vi "BenchmarkSystemDefinition.vi"(4 "Tolerance (%)":dbl=3.0 format="%#_13g", 5 "Duration (s)":dbl=30.0 format="%#_13g", 6 "Gateway IP Address (\"\": localhost)":string, 7 "Target Rate List in":dbl[](array[numeric]), 8 "error in (no error)":errorcluster, 9 "overrides files":path[](array[path]), 10 "System Definition File":path, 11 "VeriStandTestCase in":refnum<class "VeriStandTestCase.lvclass">) -> (0 "error out":errorcluster, 3 "VeriStandTestCase out":refnum<class "VeriStandTestCase.lvclass">)   [LabVIEW 2027, in "VeriStandTestCase.lvclass"]
uses:
  VeriStandTestCase.lvclass
  VeriStandTestCase.lvclass/VeriStandTestCase.ctl
  Utilities/BenchmarkInformation.ctl
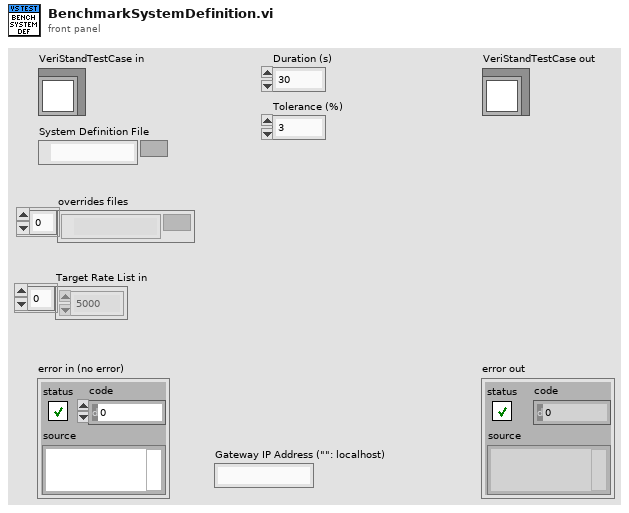
[diagram p1: front panel]
types:
  T1 = typedef "VeriStandTestCase.lvclass/BenchmarkInformation.ctl" = cluster{"Target Rate (Hz)":dbl, "Duration (s)":dbl, "Tolerance (%)":dbl, "Mean Loop Rate (Hz)":dbl, "HP Count":dbl, "Pass?":bool}
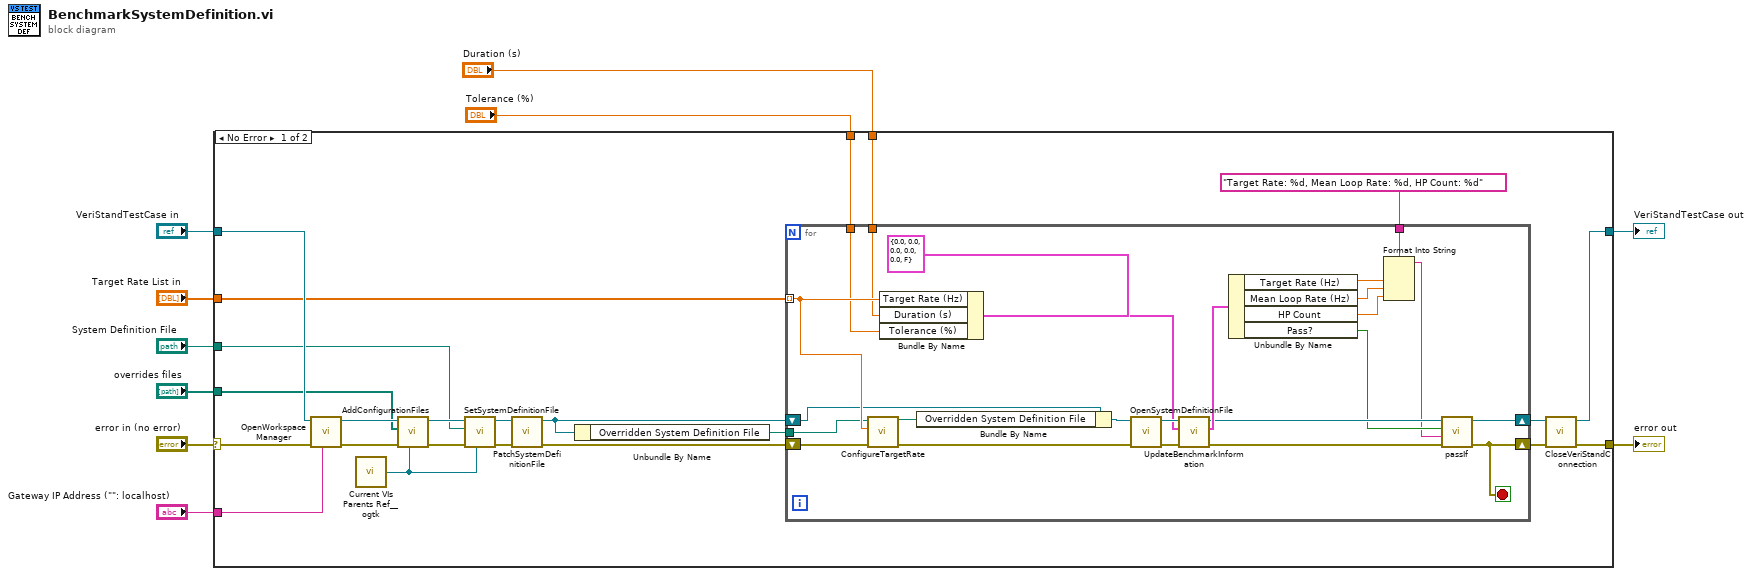
[diagram p0: block diagram]
diagram:
  n1 = case shown="No Error" "error in (no error)" {
    selector: "error in (no error)" -> [w31 w59]
    tunnel: [w33 w59] -> w9
    tunnel: [w28 w58] -> w7
    tunnel: "VeriStandTestCase in" -> [w32 w58]
    tunnel: "Gateway IP Address (\"\": localhost)" -> [w30 _]
    tunnel: "overrides files" -> [w18 _]
    tunnel: "System Definition File" -> [w17 _]
    tunnel: "Target Rate List in" -> [w26 _]
    tunnel: "Duration (s)" -> [w24 _]
    tunnel: "Tolerance (%)" -> [w23 _]
    frame No Error {
      n2 = call "OpenWorkspaceManager.vi"("Gateway IP Address (\"\": localhost)"=w30, "error in (no error)"=w31, "VeriStandTestCase in"=w32) -> ("error out"=w22:errorcluster, "VeriStandTestCase out"=w20:refnum<class "VeriStandTestCase.lvclass">)  [unwired: 7 in]
      n3 = call <userlib>:"Current VIs Parents Ref__ogtk.vi"() -> ("Calling VI's Reference"=w16:refnum<vi>)  [unwired: 2 in]
      n4 = call "AddConfigurationFiles.vi"("path root vi ref (calling vi)"=w16, "error in (no error)"=w22, "configuration files"=w18, "VeriStandTestCase in"=w20) -> ("error out"=w21:errorcluster, "VeriStandTestCase out"=w19:refnum<class "VeriStandTestCase.lvclass">)  [unwired: 6 in]
      n5 = call "SetSystemDefinitionFile.vi"("path root vi ref (calling vi)"=w16, "error in (no error)"=w21, "system definition file"=w17, "VeriStandTestCase in"=w19) -> ("error out"=w15:errorcluster, "VeriStandTestCase out"=w14:refnum<class "VeriStandTestCase.lvclass">)  [unwired: 6 in]
      n6 = call "PatchSystemDefinitionFile.vi"("error in (no error)"=w15, "VeriStand Test Case in"=w14) -> ("error out"=w13:errorcluster, "VeriStand Test Case out"=w12:refnum<class "VeriStandTestCase.lvclass">)  [unwired: 8 in]
      n7 = Unbundle By Name(w12) -> ("Overridden System Definition File"=w11:path)
      n8 = for {
        shift-right: [w48] -> w29
        shift-left: w13 -> [w56]
        shift-right: [w50] -> w27
        shift-left: w12 -> [w35]
        tunnel: w26 -> [w45] mode=indexing
        tunnel: "Target Rate: %d, Mean Loop Rate: %d, HP Count: %d" ("format string") -> [w44]
        tunnel: w24 -> [w39]
        tunnel: w23 -> [w38]
        tunnel: w11 -> [w37]
        stop <- w48 stop-if-true
        n9 = call "ConfigureTargetRate.vi"("error in (no error)"=w56, "Target Rate in"=w45, "absolute overridden system definition file in"=w37) -> ("error out"=w55:errorcluster, "absolute overridden system definition file out"=w34:path)  [unwired: 7 in]
        n10 = Bundle By Name(cluster=T1 {"Target Rate (Hz)"=0.0, "Duration (s)"=0.0, "Tolerance (%)"=0.0, "Mean Loop Rate (Hz)"=0.0, "HP Count"=0.0, "Pass?"=FALSE} ("Benchmark Information"), "Target Rate (Hz)"=w45, "Duration (s)"=w39, "Tolerance (%)"=w38) -> (w46:T1)
        n11 = Bundle By Name(cluster=w35, "Overridden System Definition File"=w34) -> (w36:refnum<class "VeriStandTestCase.lvclass">)
        n12 = call "OpenSystemDefinitionFile.vi"("error in (no error)"=w55, "VeriStand Test Case in"=w36) -> ("error out"=w57:errorcluster, "VeriStand Test Case out"=w53:refnum<class "VeriStandTestCase.lvclass">)  [unwired: 8 in]
        n13 = call "UpdateBenchmarkInformation.vi"("error in (no error)"=w57, "Benchmark Information in"=w46, "VeriStandTestCase in"=w53) -> ("error out"=w54:errorcluster, "Benchmark Information"=w52:T1, "VeriStandTestCase out"=w51:refnum<class "VeriStandTestCase.lvclass">)  [unwired: 6 in]
        n14 = Unbundle By Name(w52) -> ("Target Rate (Hz)"=w43:dbl, "Mean Loop Rate (Hz)"=w42:dbl, "HP Count"=w41:dbl, "Pass?"=w49:bool)
        n15 = Format Into String(format string=w44, w43, w42, w41) -> (resulting string=w40:string)  [unwired: 2 in, 1 out]
        n16 = call-dynamic "passIf.vi"("error in (no error)"=w54, "message (\"\")"=w40, "pass"=w49, "TestCase in"=w51) -> ("error out"=w48:errorcluster, "TestCase out"=w50:refnum<class "VeriStandTestCase.lvclass">)  [unwired: 6 in]
      }
      n17 = call-dynamic "CloseVeriStandConnection.vi"("error in (no error)"=w29, "VeriStand Test Case in"=w27) -> ("error out"=w33:errorcluster, "VeriStand Test Case out"=w28:refnum<class "VeriStandTestCase.lvclass">)  [unwired: 8 in]
    }
    frame Error {
    }
  }
  "error out" <- w9
  "VeriStandTestCase out" <- w7
